vi "Load_Zspec_param_options_SubVI.vi"(8 "error in (no error)":errorcluster, 10 "Zspecparam.txt location":path, 11 "Array in":refnum<vi>) -> (3 "Array":string[](array[string]))   [LabVIEW 2014]
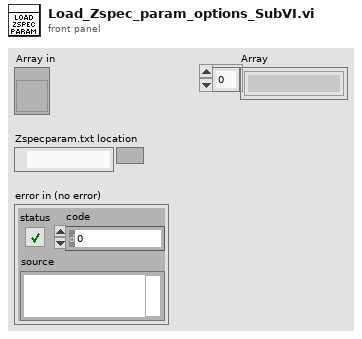
[diagram p1: front panel]
types:
  T1 = cluster{"Amplitude (mod. signal unit)":sgl, "Lockin on/off status":bool, "Backward sweep":bool, "Number of points":i32, "Channels":string[], "Parameters":string[], "Fixed parameters":string[], "Multiple sweeps configuration":cluster{"Number of Sweeps":i32, "Save all":bool}, "Initialization":cluster{"Z averaging time (s)":sgl, "Initial settling time (s)":sgl}, "Sweep Timing":cluster{"Max. slew rate (V/s)":sgl, "Settling time (s)":sgl, "Integration time (s)":sgl}, "End of Sweep":cluster{"End settling time (s)":sgl, "Z control time (s)":sgl}, "Initial Z-Offset (m)":sgl, "Sweep Distance (m)":sgl, "Channels 2":i32[], "Name":string, "Reset Z":bool, "Record final Z":bool, "Auto Retract Status":bool, "Threshold":sgl, "Auto Retract Signal Index":i32, "Auto Retract Condition":bool}[]
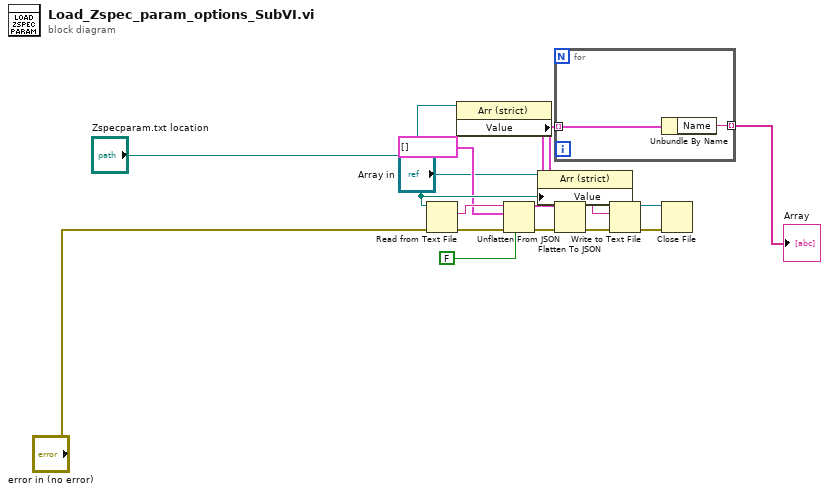
[diagram p0: block diagram]
diagram:
  n1 = Read from Text File(file (use dialog)="Zspecparam.txt location", error in="error in (no error)") -> (text=w8:string, error out=w9:errorcluster)  [unwired: 2 in, 2 out]
  n2 = property class="Arr (strict)"(reference="Array in") -> ("Value"=w13:T1)  [unwired: 1 in, 2 out]
  n3 = Unflatten From JSON(JSON string=w8, type and defaults=T1 [] ("data"), default null elements? (F)=FALSE, error in (no error)=w9) -> (value=w6:T1, error out=w3:errorcluster)  [unwired: 3 in]
  n4 = property class="Arr (strict)"(reference="Array in", "Value"=w6) -> ()  [unwired: 1 in, 2 out]
  n5 = for {
    tunnel: w6 -> [w17] mode=indexing
    tunnel: [w16] -> w5 mode=indexing
    n6 = Unbundle By Name(w17) -> ("Name"=w16:string)
  }
  "Array" <- w5
  n7 = Flatten To JSON(anything=w13, error in (no error)=w3) -> (JSON string=w12:string, 11:w14:errorcluster)  [unwired: 1 in]
  n8 = Write to Text File(file (use dialog)="Zspecparam.txt location", text=w12, error in=w14) -> (refnum out=w11:refnum<file>, error out=w10:errorcluster)  [unwired: 1 in, 1 out]
  n9 = Close File(refnum=w11, error in=w10) -> ()  [unwired: 2 out]
